vi "denglu.vi"(3 "key":string, 6 "xpswd":string, 7 "LabVIEW Web Service Request":refnum<class "Web Request.lvclass"> caption="LabVIEW Web服务请求", 8 "action":string, 10 "pswd":string, 11 "id":string) -> ()   [LabVIEW 2017]
uses:
  <vilib>/wsapi/Web Request.lvclass
panel:
  out "error":errorcluster
  out "error 1":errorcluster caption="error out 10"
  out "postdata":string caption="post数据"
  # "Web服务请求输入接线端用于调用“Web服务”选板的VI。除非不需要访问该选板，否则不要在连线板上删除这个输入接线端。"
  # "添加至连线板的每一个其他输入控件，在URL中对应于一个输入。如需在接线端模式输出（默认设置）下包含显示控件，则该显示控件必须与连线板相连。"
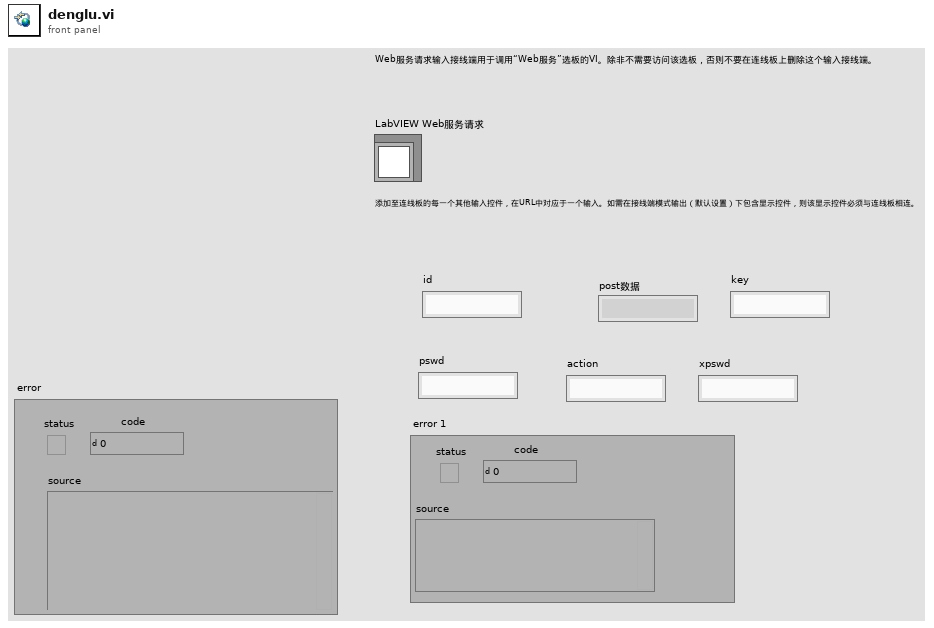
[diagram p1: front panel]
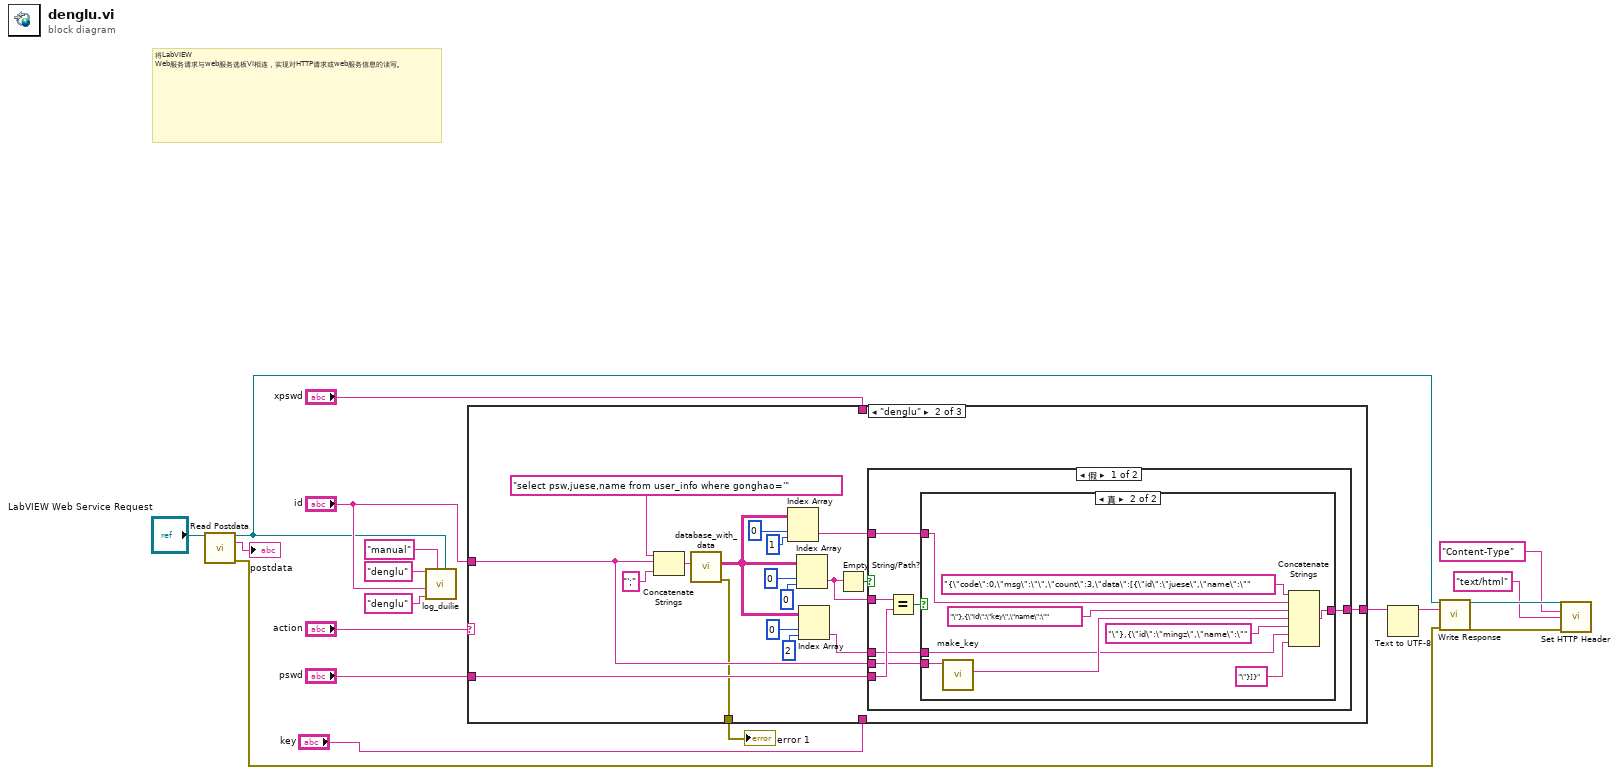
[diagram p0: block diagram]
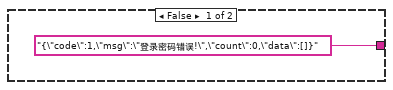
[diagram p3: hidden frame]
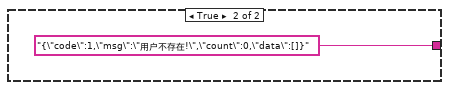
[diagram p4: hidden frame]
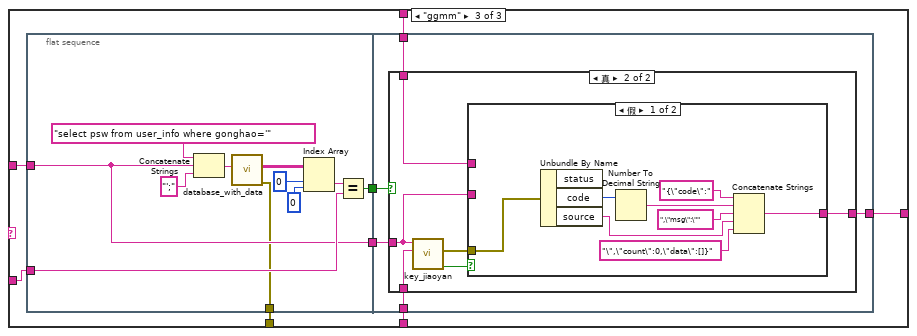
[diagram p5: hidden frame]
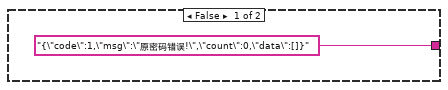
[diagram p6: hidden frame]
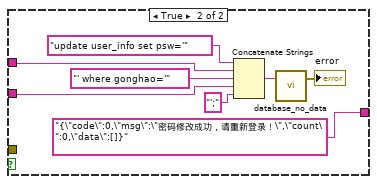
[diagram p7: hidden frame]
diagram:
  # "将LabVIEW Web服务请求与web服务选板VI相连，实现对HTTP请求或web服务信息的读写。"
  n1 = call <vilib>:"Read Postdata.vi"("LabVIEW Web Service Request"="LabVIEW Web Service Request") -> ("LabVIEW Web Service Request out"=w5:refnum<class "Web Request.lvclass">, "postdata"=→"postdata":string, "error out"=w15:errorcluster)  [unwired: 12 in]
  n2 = call "log_duilie.vi"("LabVIEW Web Service Request"=w5, "type"="manual", "action"="denglu", "user"="id", "yw"="denglu") -> ()  [unwired: 7 in]
  n3 = case shown="\"denglu\"" "action" {
    tunnel: "id" -> [_ w27 w63]
    tunnel: "pswd" -> [_ w26 w62]
    tunnel: [_ w25 w60] -> w4
    tunnel: "xpswd" -> [_ _ w59]
    tunnel: [_ w24 w57] -> w2
    tunnel: "key" -> [_ _ w56]
    frame "假", Default {
    }
    frame "denglu" {
      n4 = Concatenate Strings("select psw,juese,name from user_info where gonghao='" ("Command Text"), w27, "';" ("字符串")) -> (w37:string)
      n5 = call "database_with_data.vi"("input"=w37) -> ("error"=w24:errorcluster, "Data"=w21:string[][])  [unwired: 9 in]
      n6 = Index Array(array=w21, index (row)=0 ("索引 (行)"), index (col)=1 ("禁用的索引 (列)")) -> (element=w28:string)
      n7 = Index Array(array=w21, index (row)=0 ("索引 (行)"), index (col)=0 ("禁用的索引 (列)")) -> (element=w31:string)
      n8 = Index Array(array=w21, index (row)=0 ("索引 (行)"), index (col)=2 ("禁用的索引 (列)")) -> (element=w20:string)
      n9 = Empty String/Path?(string/path=w31) -> (empty?=w32:bool)
      n10 = case shown="假" w32 {
        tunnel: w26 -> [w44 _]
        tunnel: w31 -> [w43 _]
        tunnel: w28 -> [w41 _]
        tunnel: [w40 "{\"code\":1,\"msg\":\"用户不存在!\",\"count\":0,\"data\":[]}" ("字符串")] -> w25
        tunnel: w27 -> [w39 _]
        tunnel: w20 -> [w38 _]
        frame False {
          n11 = Equal?(x=w43, y=w44) -> (x = y?=w42:bool)
          n12 = case shown="真" w42 {
            tunnel: w41 -> [_ w52]
            tunnel: ["{\"code\":1,\"msg\":\"登录密码错误!\",\"count\":0,\"data\":[]}" ("字符串") w48] -> w40
            tunnel: w39 -> [_ w54]
            tunnel: w38 -> [_ w46]
            frame False {
            }
            frame True {
              n13 = call "make_key.vi"("gonghao"=w54) -> ("key_out"=w50:string)  [unwired: 10 in]
              n14 = Concatenate Strings("{\"code\":0,\"msg\":\"\",\"count\":3,\"data\":[{\"id\":\"juese\",\"name\":\"" ("字符串"), w52, "\"},{\"id\":\"key\",\"name\":\"" ("字符串"), w50, "\"},{\"id\":\"mingz\",\"name\":\"" ("字符串"), w46, "\"}]}" ("字符串")) -> (w48:string)
            }
          }
        }
        frame True {
        }
      }
    }
    frame "ggmm" {
      n15 = flat-sequence {
        tunnel: w63 -> [w65]
        tunnel: w62 -> [w67]
        tunnel: [w66] -> w61
        tunnel: [w65] -> w58
        tunnel: [w64] -> w57
        tunnel: w61 -> [w79]
        tunnel: [w78] -> w60
        tunnel: w59 -> [w77]
        tunnel: w58 -> [w76]
        tunnel: w56 -> [w75]
        frame #0 {
          n16 = Concatenate Strings("select psw from user_info where gonghao='" ("Command Text"), w65, "';" ("字符串")) -> (w74:string)
          n17 = call "database_with_data.vi"("input"=w74) -> ("error"=w64:errorcluster, "Data"=w68:string[][])  [unwired: 9 in]
          n18 = Index Array(array=w68, index (row)=0 ("索引 (行)"), index (col)=0 ("禁用的索引 (列)")) -> (element=w69:string)
          n19 = Equal?(x=w69, y=w67) -> (x = y?=w66:bool)
        }
        frame #1 {
          n20 = case shown="真" w79 {
            tunnel: ["{\"code\":1,\"msg\":\"原密码错误!\",\"count\":0,\"data\":[]}" ("字符串") w86] -> w78
            tunnel: w77 -> [_ w85]
            tunnel: w76 -> [_ w84]
            tunnel: w75 -> [_ w83]
            frame False {
            }
            frame True {
              n21 = call "key_jiaoyan.vi"("key_client"=w83, "gonghao"=w84) -> ("jy"=w82:bool, "error"=w81:errorcluster)  [unwired: 8 in]
              n22 = case shown="假" w82 {
                tunnel: [w88 "{\"code\":0,\"msg\":\"密码修改成功，请重新登录！\",\"count\":0,\"data\":[]}" ("字符串")] -> w86
                tunnel: w85 -> [_ w97]
                tunnel: w84 -> [_ w95]
                tunnel: w81 -> [w87 _]
                frame False {
                  n23 = Unbundle By Name(w87) -> ("code"=w92:i32, "source"=w94:string)  [unwired: 1 out]
                  n24 = Number To Decimal String(number=w92) -> (decimal integer string=w93:string)  [unwired: 1 in]
                  n25 = Concatenate Strings("{\"code\":" ("字符串"), w93, ",\"msg\":\"" ("字符串"), w94, "\",\"count\":0,\"data\":[]}" ("字符串")) -> (w88:string)
                }
                frame True {
                  n26 = Concatenate Strings("update user_info set psw='" ("格式字符串"), w97, "' where gonghao='" ("字符串"), w95, "';" ("字符串")) -> (w101:string)
                  n27 = call "database_no_data.vi"("input"=w101) -> ("error"=→"error":errorcluster)  [unwired: 2 in]
                }
              }
            }
          }
        }
      }
    }
  }
  "error 1" <- w2
  n28 = Text to UTF-8(11:w4) -> (3:w13:string)  [unwired: 2 in, 1 out]
  n29 = call <vilib>:"Write Response.vi"("LabVIEW Web Service Request"=w5, "response string"=w13, "error in (no error)"=w15) -> ("LabVIEW Web Service Request out"=w19:refnum<class "Web Request.lvclass">, "error out"=w18:errorcluster)  [unwired: 11 in]
  n30 = call <vilib>:"Set HTTP Header.vi"("LabVIEW Web Service Request"=w19, "header"="Content-Type", "header value"="text/html", "error in (no error)"=w18) -> ()  [unwired: 10 in, 2 out]
